vi "main.vi"   [LabVIEW 2019]
panel:
  # "Desktop App"
types:
  T1 = typedef "Queues.ctl" = cluster{"GUIOutput":refnum<queue>, "AnalyzedVibrationsData":refnum<queue>, "Command":refnum<queue>, "TDMSAnalyzerData":refnum<queue>, "DataToSave":refnum<queue>}
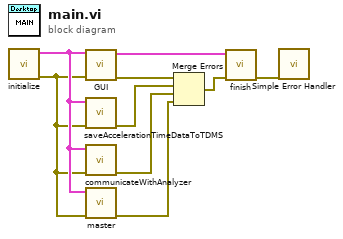
[diagram p0: block diagram]
diagram:
  n1 = call "initialize.vi"() -> ("ErrorOut"=w1:errorcluster, "Queues"=w3:T1)  [unwired: 10 in]
  n2 = call "GUI.vi"("ErrorIn"=w1, "QueuesIn"=w3) -> ("ErrorOut"=w9:errorcluster, "QueuesOut"=w4:T1)  [unwired: 8 in]
  n3 = call "saveAccelerationTimeDataToTDMS.vi"("ErrorIn"=w1, "QueuesIn"=w3) -> ("ErrorOut"=w6:errorcluster)  [unwired: 8 in, 1 out]
  n4 = call "communicateWithAnalyzer.vi"("ErrorIn"=w1, "QueuesIn"=w3) -> ("ErrorOut"=w5:errorcluster)  [unwired: 8 in, 1 out]
  n5 = call "master.vi"("ErrorIn"=w1, "QueuesIn"=w3) -> ("ErrorOut"=w2:errorcluster)  [unwired: 8 in, 1 out]
  n6 = Merge Errors(w9, w6, w5, w2) -> (w7:errorcluster)
  n7 = call "finish.vi"("ErrorIn"=w7, "Queues"=w4) -> ("ErrorOut"=w8:errorcluster)  [unwired: 9 in]
  n8 = call <vilib>:"Simple Error Handler.vi"("error in (no error)"=w8) -> ()  [unwired: 4 in, 5 out]
